vi "Teleop.vi"(10 "Match Info":T1={"Autonomous Elapsed Seconds"=0.0, "TeleOp Elapsed Seconds"=0.0, "Disabled Elapsed Seconds"=0.0, "Visited Autonomous"=FALSE, "Visited TeleOp"=FALSE, "Visited Disabled"=FALSE, "Autonomous Settings"={"Autonomous Style"=enum."Independent", "VI Refnum"=refnum}}, 11 "Call Context":T2) -> ()   [LabVIEW 2016]
doc: "This VI is called for each TeleOp packet received from the DS where the robot is not disabled. It is often used to read from the joysticks and update I/O or to update setpoints for timed control loops. It should complete and return within 20 milliseconds or it may miss DS packets."
uses:
  <vilib>/Rock Robotics/WPI/DriverStation/WPI_DriverStationDerivedRobotMode.ctl
  <vilib>/Rock Robotics/WPI/DriverStation/WPI_DriverStationMatch Info.ctl
  <vilib>/Rock Robotics/WPI/Solenoid/WPI_SolenoidValue.ctl
  <vilib>/Rock Robotics/Network Tables/NT Read Boolean.vi
  <vilib>/Rock Robotics/Network Tables/NT Read Number.vi
  <vilib>/Rock Robotics/WPI/Utilities/WPI_GetSetVariantRefNum.vi
  <vilib>/Rock Robotics/WPI/Solenoid/WPI_SolenoidSetEnum.vi
  <vilib>/Rock Robotics/WPI/Solenoid/Deprecated/WPI_SolenoidGetBool.vi
  <vilib>/Rock Robotics/Network Tables/NT Write Boolean.vi
panel:
  in  "Reset":bool
  out "Teleop Time Elipsed":dbl
  in  "Quand arreter compresseur":dbl
  out "Droit":dbl
  out "Gauche":dbl
  out "Sample Slider 0":dbl(slide) scale=0.0..5.0
  out "Sample Boolean 1":bool
  out "Sample Boolean 0":bool
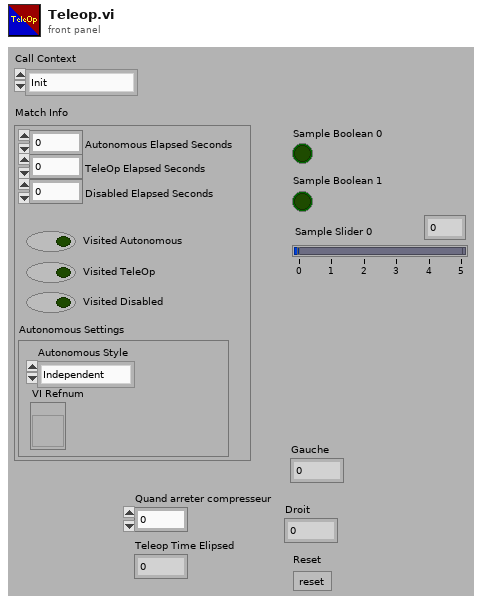
[diagram p1: front panel]
types:
  T1 = typedef "WPI_DriverStationMatch Info.ctl" = cluster{"Autonomous Elapsed Seconds":dbl, "TeleOp Elapsed Seconds":dbl, "Disabled Elapsed Seconds":dbl, "Visited Autonomous":bool, "Visited TeleOp":bool, "Visited Disabled":bool, "Autonomous Settings":cluster{"Autonomous Style":enum16{"Iterative", "Independent"}, "VI Refnum":refnum<vi>}}
  T2 = typedef "WPI_DriverStationDerivedRobotMode.ctl" = enum16{"Init", "Execute", "Stop"}
  T3 = typedef "WPI_SolenoidValue.ctl" = enum16{"Off", "On", "Forward", "Reverse"}
  T4 = typedef "WPI_EncoderDevRef.ctl" = cluster{"DevStatus":errorcluster, "EncoderIndex":T5, "CounterIndex":T6, "DistancePerCount":dbl, "Decoding Type":T7}
  T5 = typedef "FPGA_EncoderIdx.ctl" = enum8{"Enc 0", "Enc 1", "Enc 2", "Enc 3", "Enc 4", "Enc 5", "Enc 6", "Enc 7", "Invalid"}
  T6 = typedef "FPGA_CounterCtrSystemIndex.ctl" = enum8{"Ctr 0", "Ctr 1", "Ctr 2", "Ctr 3", "Ctr 4", "Ctr 5", "Ctr 6", "Ctr 7", "Invalid"}
  T7 = typedef "WPI_EncoderType.ctl" = enum16{"1x", "2x", "4x"}
  T8 = typedef "WPI_SolenoidDevRef.ctl" = cluster{"DevStatus":errorcluster, "Pneumatics Control Module":u8, "Forward Solenoid Channel":T9, "Reverse Solenoid Channel":T9}
  T9 = typedef "WPI_SolenoidChannel.ctl" = enum8{"Solenoid 0", "Solenoid 1", "Solenoid 2", "Solenoid 3", "Solenoid 4", "Solenoid 5", "Solenoid 6", "Solenoid 7", "Invalid"}
  T10 = typedef "WPI_JoystickDevRef.ctl" = cluster{"Device":T11}
  T11 = typedef "WPI_JoystickDeviceEnum.ctl" = enum16{"USB 0", "USB 1", "USB 2", "USB 3", "USB 4", "USB 5"}
  T12 = cluster{"Axes[0]":dbl, "Axes[1]":dbl, "Axes[2]":dbl, "Axes[3]":dbl, "Axes[4]":dbl, "Axes[5]":dbl, "Axes[6]":dbl, "Axes[7]":dbl, "Axes[8]":dbl}
  T13 = cluster{"Buttons[0]":bool, "Buttons[1]":bool, "Buttons[2]":bool, "Buttons[3]":bool, "Buttons[4]":bool, "Buttons[5]":bool, "Buttons[6]":bool, "Buttons[7]":bool, "Buttons[8]":bool}
  T14 = typedef "WPI_CompressorDevRef.ctl" = cluster{"DevStatus":errorcluster, "Pneumatics Control Module":u8}
  T15 = typedef "WPI_MotorControlDeviceRef.ctl" = cluster{"DeviceStatus":errorcluster, "Type":T16, "PWM":cluster{"PWM Channel":T17, "DeadBand":T18}, "CAN":cluster{"Device Number":u8, "SetOutput VI Ref":variant, "GetOutput VI Ref":variant, "Enable VI Ref":variant, "Disable VI Ref":variant, "Data":variant}, "Invert":bool}
  T16 = typedef "WPI_MotorControlType.ctl" = enum16{"PWM", "CAN"}
  T17 = typedef "FPGA_DIOPWMChannel.ctl" = enum8{"PWM 0", "PWM 1", "PWM 2", "PWM 3", "PWM 4", "PWM 5", "PWM 6", "PWM 7", "PWM 8", "PWM 9", "PWM MXP 0", "PWM MXP 1", "PWM MXP 2", "PWM MXP 3", "PWM MXP 4", "PWM MXP 5", "PWM MXP 6", "PWM MXP 7", "PWM MXP 8", "PWM MXP 9", "Invalid"}
  T18 = typedef "WPI_PWMDeadband.ctl" = cluster{"Name":string, "maxPositivePwm":i32, "minPositivePwm":i32, "centerPwm":i32, "maxNegativePwm":i32, "minNegativePwm":i32, "angularRange":u16}
  T19 = typedef "WPI_RobotDriveDevRef.ctl" = cluster{"DevStatus":errorcluster, "Motors[]":T15[], "Square Inputs":bool, "Max Output":dbl}
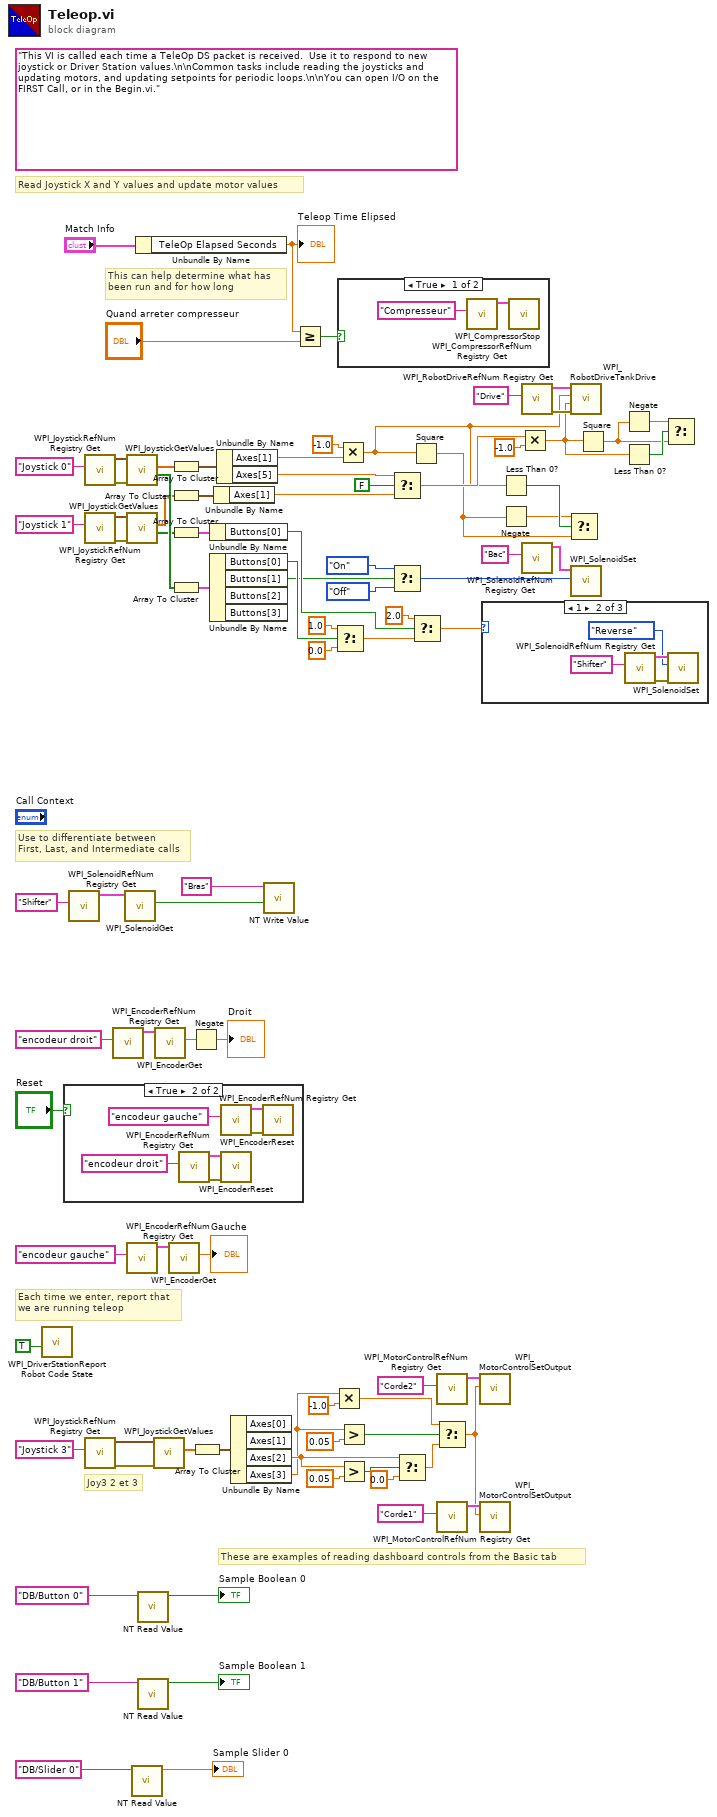
[diagram p0: block diagram]
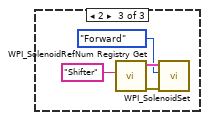
[diagram p5: hidden frame]
diagram:
  (unwired) "This VI is called each time a TeleOp DS packet is received.  Use it to respond to new joystick or Driver Station values.\n\nCommon tasks include reading the joysticks and updating motors, and updating setpoints for periodic loops.\n\nYou can open I/O on the FIRST Call, or in the Begin.vi."
  # "Joy3 2 et 3"
  # "These are examples of reading dashboard controls from the Basic tab"
  # "Each time we enter, report that\nwe are running teleop"
  # "Use to differentiate between\nFirst, Last, and Intermediate calls"
  # "This can help determine what has\nbeen run and for how long"
  # "Read Joystick X and Y values and update motor values"
  n1 = call <vilib>:"WPI_DriverStationReport Robot Code State.vi"("TeleOp"=TRUE ("Autonomous")) -> ()  [unwired: 10 in, 1 out]
  n2 = case shown="True" "Reset" {
    frame False {
    }
    frame True {
      n3 = call <vilib>:"WPI_EncoderRefNum Registry Get.vi"("refnum name"="encodeur droit") -> ("error out"=w91:errorcluster, "EncoderDevRef"=w92:T4)  [unwired: 9 in]
      n4 = call <vilib>:"WPI_EncoderRefNum Registry Get.vi"("refnum name"="encodeur gauche") -> ("error out"=w90:errorcluster, "EncoderDevRef"=w89:T4)  [unwired: 9 in]
      n5 = call <vilib>:"WPI_EncoderReset.vi"("error in (no error)"=w91, "EncoderDevRef"=w92) -> ()  [unwired: 8 in, 2 out]
      n6 = call <vilib>:"WPI_EncoderReset.vi"("error in (no error)"=w90, "EncoderDevRef"=w89) -> ()  [unwired: 8 in, 2 out]
    }
  }
  n7 = call <vilib>:"WPI_SolenoidRefNum Registry Get.vi"("refnum name"="Shifter") -> ("SolenoidDevRef"=w20:T8)  [unwired: 9 in, 1 out]
  n8 = call <vilib>:"WPI_JoystickRefNum Registry Get.vi"("refnum name"="Joystick 0") -> ("error out"=w77:errorcluster, "JoystickDevRef"=w76:T10)  [unwired: 9 in]
  n9 = call <vilib>:"WPI_JoystickRefNum Registry Get.vi"("refnum name"="Joystick 1") -> ("error out"=w46:errorcluster, "JoystickDevRef"=w45:T10)  [unwired: 9 in]
  n10 = call <vilib>:"WPI_JoystickRefNum Registry Get.vi"("refnum name"="Joystick 3") -> ("error out"=w59:errorcluster, "JoystickDevRef"=w60:T10)  [unwired: 1 in, 8 out]
  n11 = call <vilib>:"WPI_EncoderRefNum Registry Get.vi"("refnum name"="encodeur droit") -> ("EncoderDevRef"=w56:T4)  [unwired: 9 in, 1 out]
  n12 = call-poly <vilib>:"WPI_SolenoidGet.vi"("SolenoidDevRef"=w20) -> ("Value"=w19:bool)  [unwired: 8 in, 2 out]
  n13 = call <vilib>:"WPI_JoystickGetValues.vi"("error in (no error)"=w77, "JoystickDevRef"=w76) -> ("Buttons"=w72:bool[], "Axes"=w75:dbl[])  [unwired: 5 in, 3 out]
  n14 = call <vilib>:"WPI_JoystickGetValues.vi"("error in (no error)"=w46, "JoystickDevRef"=w45) -> ("Buttons"=w37:bool[], "Axes"=w44:dbl[])  [unwired: 5 in, 3 out]
  n15 = call <vilib>:"WPI_EncoderRefNum Registry Get.vi"("refnum name"="encodeur gauche") -> ("EncoderDevRef"=w57:T4)  [unwired: 9 in, 1 out]
  n16 = call-poly <vilib>:"NT Read Value.vi"("Name"="DB/Slider 0" ("refnum name")) -> ("Numeric"=→"Sample Slider 0":dbl)  [unwired: 9 in, 1 out]
  n17 = Unbundle By Name("Match Info") -> ("TeleOp Elapsed Seconds"=w50:dbl)
  "Teleop Time Elipsed" <- w50
  n18 = call-poly <vilib>:"NT Read Value.vi"("Name"="DB/Button 0" ("refnum name")) -> ("Boolean"=→"Sample Boolean 0":bool)  [unwired: 9 in, 1 out]
  n19 = call-poly <vilib>:"NT Read Value.vi"("Name"="DB/Button 1" ("refnum name")) -> ("Boolean"=→"Sample Boolean 1":bool)  [unwired: 9 in, 1 out]
  n20 = call <vilib>:"WPI_JoystickGetValues.vi"("error in (no error)"=w59, "JoystickDevRef"=w60) -> ("Axes"=w16:dbl[])  [unwired: 5 in, 4 out]
  n21 = call <vilib>:"WPI_EncoderGet.vi"("EncoderDevRef"=w56) -> ("Distance"=w40:dbl)  [unwired: 5 in, 5 out]
  n22 = call <vilib>:"WPI_EncoderGet.vi"("EncoderDevRef"=w57) -> ("Distance"=→"Gauche":dbl)  [unwired: 5 in, 5 out]
  n23 = Array To Cluster(array=w75) -> (cluster=w74:T12)
  n24 = Array To Cluster(array=w44) -> (cluster=w43:T12)
  n25 = Array To Cluster(array=w37) -> (cluster=w36:T13)
  n26 = Array To Cluster(array=w72) -> (cluster=w38:T13)
  n27 = Negate(x=w40) -> (-x=→"Droit":dbl)
  n28 = Array To Cluster(array=w16) -> (cluster=w58:T12)
  n29 = Unbundle By Name(w36) -> ("Buttons[0]"=w34:bool)
  n30 = Unbundle By Name(w38) -> ("Buttons[0]"=w35:bool, "Buttons[1]"=w17:bool)  [unwired: 2 out]
  n31 = Unbundle By Name(w43) -> ("Axes[1]"=w31:dbl)
  n32 = Unbundle By Name(w74) -> ("Axes[1]"=w49:dbl, "Axes[5]"=w32:dbl)
  n33 = Unbundle By Name(w58) -> ("Axes[2]"=w11:dbl, "Axes[3]"=w7:dbl)  [unwired: 2 out]
  n34 = call-poly <vilib>:"NT Write Value.vi"("Boolean"=w19, "Name"="Bras") -> ()  [unwired: 9 in, 1 out]
  n35 = Greater Or Equal?(x=w50, y="Quand arreter compresseur") -> (x >= y?=w51:bool)
  n36 = Multiply(x=w7, y=-1.0) -> (x*y=w6:dbl)
  n37 = Select(t=1.0, s=w35, f=0.0) -> (s? t:f=w70:dbl)
  n38 = case shown="True" w51 {
    frame True {
      n39 = call <vilib>:"WPI_CompressorRefNum Registry Get.vi"("refnum name"="Compresseur") -> ("CompressorDevRef"=w96:T14)  [unwired: 9 in, 1 out]
      n40 = call <vilib>:"WPI_CompressorStop.vi"("CompressorDevRef"=w96) -> ()  [unwired: 9 in, 2 out]
    }
    frame False {
    }
  }
  n41 = Multiply(x=-1.0, y=w49) -> (x*y=w23:dbl)
  n42 = Greater?(x=w7, y=0.05) -> (0:w9:bool)
  n43 = Greater?(x=w11, y=0.05) -> (0:w13:bool)
  n44 = Select(t=w32, s=FALSE, f=w31) -> (s? t:f=w33:dbl)
  n45 = Select(t=WPI_SolenoidValue."On" ("Value"), s=w17, f=WPI_SolenoidValue."Off" ("Value")) -> (s? t:f=w62:T3)
  n46 = Select(t=w11, s=w13, f=0.0) -> (s? t:f=w10:dbl)
  n47 = Square(x=w23) -> (x^2=w27:dbl)
  n48 = Select(t=2.0, s=w34, f=w70) -> (s? t:f=w67:dbl)
  n49 = call <vilib>:"WPI_MotorControlRefNum Registry Get.vi"("refnum name"="Corde2") -> ("MotorControlDevRef"=w5:T15)  [unwired: 9 in, 1 out]
  n50 = Select(t=w6, s=w9, f=w10) -> (s? t:f=w1:dbl)
  n51 = call <vilib>:"WPI_MotorControlRefNum Registry Get.vi"("refnum name"="Corde1") -> ("MotorControlDevRef"=w4:T15)  [unwired: 9 in, 1 out]
  n52 = call <vilib>:"WPI_MotorControlSetOutput.vi"("Output"=w1, "MotorControlDevRef"=w5) -> ()  [unwired: 7 in, 3 out]
  n53 = call <vilib>:"WPI_MotorControlSetOutput.vi"("Output"=w1, "MotorControlDevRef"=w4) -> ()  [unwired: 7 in, 3 out]
  n54 = case shown="1" w67 {
    frame 0, Default {
    }
    frame 1 {
      n55 = call <vilib>:"WPI_SolenoidRefNum Registry Get.vi"("refnum name"="Shifter") -> ("error out"=w99:errorcluster, "SolenoidDevRef"=w98:T8)  [unwired: 9 in]
      n56 = call-poly <vilib>:"WPI_SolenoidSet.vi"("error in (no error)"=w99, "Value"=WPI_SolenoidValue."Reverse", "SolenoidDevRef"=w98) -> ()  [unwired: 7 in, 2 out]
    }
    frame 2 {
      n57 = call <vilib>:"WPI_SolenoidRefNum Registry Get.vi"("refnum name"="Shifter") -> ("error out"=w103:errorcluster, "SolenoidDevRef"=w102:T8)  [unwired: 9 in]
      n58 = call-poly <vilib>:"WPI_SolenoidSet.vi"("error in (no error)"=w103, "Value"=WPI_SolenoidValue."Forward", "SolenoidDevRef"=w102) -> ()  [unwired: 7 in, 2 out]
    }
  }
  n59 = Less Than 0?(x=w23) -> (x < 0?=w29:bool)
  n60 = Negate(x=w27) -> (-x=w28:dbl)
  n61 = Multiply(x=w33, y=-1.0) -> (x*y=w22:dbl)
  n62 = call <vilib>:"WPI_RobotDriveRefNum Registry Get.vi"("refnum name"="Drive") -> ("error out"=w80:errorcluster, "RobotDriveDevRef"=w79:T19)  [unwired: 9 in]
  n63 = call <vilib>:"WPI_SolenoidRefNum Registry Get.vi"("refnum name"="Bac") -> ("SolenoidDevRef"=w63:T8)  [unwired: 9 in, 1 out]
  n64 = Select(t=w28, s=w29, f=w27) -> ()  [unwired: 1 out]
  n65 = call <vilib>:"WPI_RobotDriveTankDrive.vi"("error in (no error)"=w80, "Right axis value"=w22, "Left axis value"=w23, "RobotDriveDevRef"=w79) -> ()  [unwired: 5 in, 3 out]
  n66 = call-poly <vilib>:"WPI_SolenoidSet.vi"("Value"=w62, "SolenoidDevRef"=w63) -> ()  [unwired: 8 in, 2 out]
  n67 = Square(x=w22) -> (x^2=w25:dbl)
  n68 = Negate(x=w25) -> (-x=w24:dbl)
  n69 = Less Than 0?(x=w22) -> (x < 0?=w26:bool)
  n70 = Select(t=w24, s=w26, f=w25) -> ()  [unwired: 1 out]
